vi "Load Config.vi"(7 "Name Delimiter":string, 8 "error in (no error)":errorcluster, 11 "Config-JSON in":refnum<class "Config-JSON.lvclass">) -> (0 "error out":errorcluster, 2 "Elements":refnum<class "Config Element.lvclass">[](array[class]), 3 "Config-JSON out":refnum<class "Config-JSON.lvclass">)   [LabVIEW 2020, in "CDM-Config.lvlib" / "Config-JSON.lvclass"]
uses:
  Config-JSON.lvclass
  Config Element/Config Element.lvclass
  Config-JSON.lvclass/Config-JSON.ctl
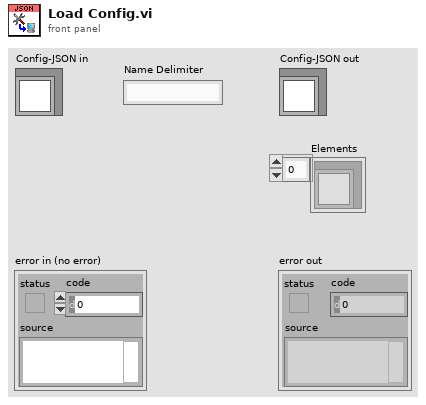
[diagram p1: front panel]
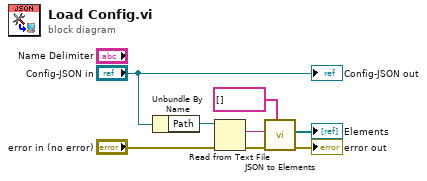
[diagram p0: block diagram]
diagram:
  n1 = Unbundle By Name("Config-JSON in") -> ("Path"=w7:path)
  n2 = Read from Text File(file (use dialog)=w7, error in="error in (no error)") -> (text=w5:string, error out=w4:errorcluster)  [unwired: 2 in, 2 out]
  n3 = call "JSON to Elements.vi"("Hierarchy"=string[] [] ("Parent Hierarchy"), "error in (no error)"=w4, "JSON"=w5) -> ("error out"=→"error out":errorcluster, "Elements"=→"Elements":refnum<class "Config Element.lvclass">[])  [unwired: 7 in]
  "Config-JSON out" <- "Config-JSON in"
